vi "calcOffsetTime.vi"(4 "Hour Offset":i32) -> (1 "currentTimeOffset":string)   [LabVIEW 2013]
doc: "this subVI inputs an offset to alter the current hour and returns the offsetTime string"
panel:
  out "Second":string
  out "Hour":string
  out "Minute":string
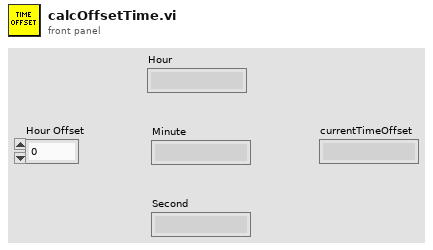
[diagram p1: front panel]
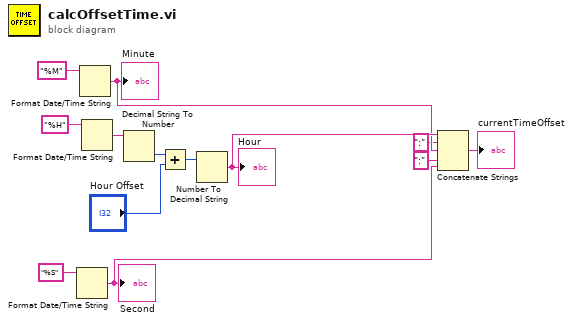
[diagram p0: block diagram]
diagram:
  n1 = Format Date/Time String(time format string (%c)="%S") -> (date/time string=w4:string)  [unwired: 2 in]
  "Second" <- w4
  n2 = Format Date/Time String(time format string (%c)="%M") -> (date/time string=w5:string)  [unwired: 2 in]
  "Minute" <- w5
  n3 = Format Date/Time String(time format string (%c)="%H") -> (date/time string=w10:string)  [unwired: 2 in]
  n4 = Decimal String To Number(string=w10) -> (number=w9:i32)  [unwired: 2 in, 1 out]
  n5 = Add(x=w9, y="Hour Offset") -> (x+y=w7:i32)
  n6 = Number To Decimal String(number=w7) -> (decimal integer string=w6:string)  [unwired: 1 in]
  "Hour" <- w6
  n7 = Concatenate Strings(w6, ":" ("string"), w5, ":" ("string"), w4) -> (→"currentTimeOffset":string)
